vi "convert area percentage to time percentage for blanking.vi"(11 "areapercentage":dbl=20.0) -> (3 "timepercentage":dbl)   [LabVIEW 2012]
doc: "SciScan 1.2 160622"
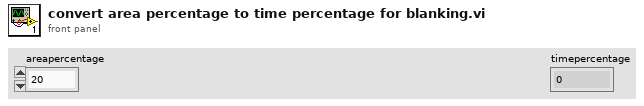
[diagram p1: front panel]
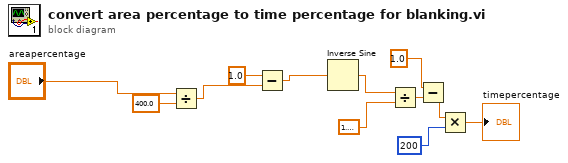
[diagram p0: block diagram]
diagram:
  n1 = Divide(x="areapercentage", y=400.0) -> (x/y=w10:dbl)
  n2 = Subtract(x=1.0, y=w10) -> (x-y=w8:dbl)
  n3 = Inverse Sine(1:w8) -> (0:w7:dbl)
  n4 = Divide(x=w7, y=1.5707963267948966) -> (x/y=w5:dbl)
  n5 = Subtract(x=1.0, y=w5) -> (x-y=w2:dbl)
  n6 = Multiply(x=w2, y=200) -> (x*y=→"timepercentage":dbl)
